vi "Create New System Definition.vi"(8 "error in (no error)":errorcluster, 9 "Settings":T2, 11 "path":path) -> (0 "error out":errorcluster, 2 "System Node Paths":T1, 3 "SysDef Ref":T3)   [LabVIEW 2019, in "Simple SysDef API.lvlib"]
uses:
  <userlib>/SimpleSysDef/Simple SysDef API.lvlib
  <userlib>/SimpleSysDef/_SubVIs/System Definition Reference.ctl
  NationalInstruments.VeriStand.SystemDefinitionAPI
  <userlib>/SimpleSysDef/_SubVIs/Create New System Definition_Settings.ctl
  <userlib>/SimpleSysDef/_SubVIs/System Node Paths.ctl
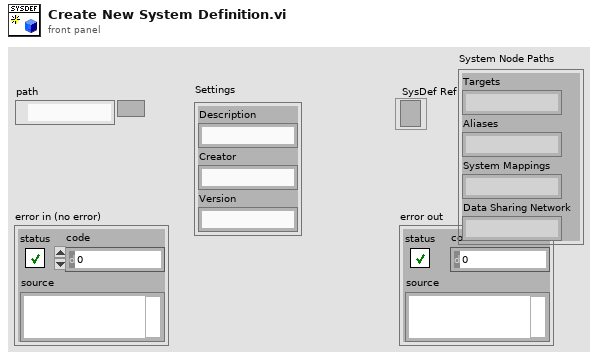
[diagram p1: front panel]
types:
  T1 = typedef "Simple SysDef API.lvlib/System Node Paths.ctl" = cluster{"Targets":string, "Aliases":string, "System Mappings":string, "Data Sharing Network":string}
  T2 = typedef "Simple SysDef API.lvlib/Create New System Definition_Settings.ctl" = cluster{"Description":string, "Creator":string, "Version":string}
  T3 = typedef "Simple SysDef API.lvlib/System Definition Reference.ctl" = refnum<k24>
  T4 = cluster{"[0]":string, "[1]":string, "[2]":string, "[3]":string}
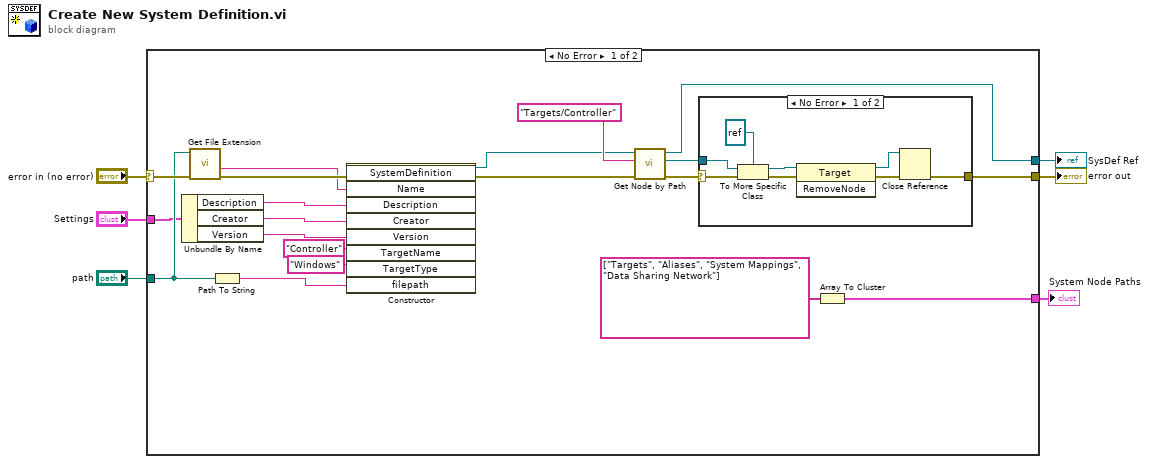
[diagram p0: block diagram]
diagram:
  n1 = case shown="No Error" "error in (no error)" {
    selector: "error in (no error)" -> [w23 w36]
    tunnel: "path" -> [w21 _]
    tunnel: [w13 w36] -> w5
    tunnel: [w12 _] -> w4
    tunnel: "Settings" -> [w19 _]
    tunnel: [w7 _] -> w1
    frame No Error {
      n2 = Unbundle By Name(w19) -> ("Description"=w18:string, "Creator"=w17:string, "Version"=w16:string)
      n3 = call <vilib>:"Get File Extension.vi"("error in (no error)"=w23, "file"=w21) -> ("error out"=w22:errorcluster, "filename without extension"=w20:string)  [unwired: 5 in, 3 out]
      n4 = Path To String(path=w21) -> (string=w26:string)
      n5 = constructor class="SystemDefinition"(error in=w22, "Name"=w20, "Description"=w18, "Creator"=w17, "Version"=w16, "TargetName"="Controller", "TargetType"="Windows", "filepath"=w26) -> (reference out=w9:refnum<k24>, error out=w10:errorcluster)  [unwired: 2 in, 8 out]
      n6 = call <userlib>:"Get Node by Path.vi"("error in (no error)"=w10, "System Definition Node Path"="Targets/Controller", "SysDef Ref"=w9) -> ("error out"=w14:errorcluster, "Node Ref"=w11:refnum<k24>, "SysDef Ref Out"=w12:T3)  [unwired: 6 in]
      n7 = case shown="No Error" w14 {
        selector: w14 -> [w33 w35]
        tunnel: [w27 w35] -> w13
        tunnel: w11 -> [w32 _]
        frame No Error {
          n8 = To More Specific Class(target class=refnum<k24> refnum ("Node Ref"), reference=w32, error in=w33) -> (specific class reference=w31:refnum<k24>, error out=w30:errorcluster)
          n9 = invoke class="Target" method="RemoveNode"(reference=w31, error in=w30) -> (reference out=w28:refnum<k24>, error out=w29:errorcluster)  [unwired: 1 in, 1 out]
          n10 = Close Reference(reference=w28, error in (no error)=w29) -> (error out=w27:errorcluster)
        }
        frame Error {
        }
      }
      n11 = Array To Cluster(array=string[] ["Targets", "Aliases", "System Mappings", "Data Sharing Network"]) -> (cluster=w7:T4)
    }
    frame Error {
    }
  }
  "error out" <- w5
  "SysDef Ref" <- w4
  "System Node Paths" <- w1
